vi "Normal to HEX string.vi"(1 "input normal string":string="0100") -> (0 "output HEX string":string)   [LabVIEW 2023]
panel:
  out "reversed":string
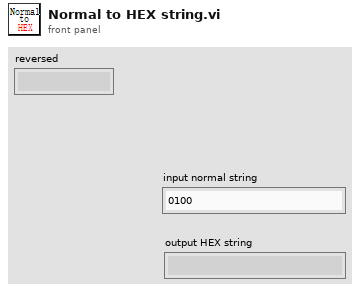
[diagram p1: front panel]
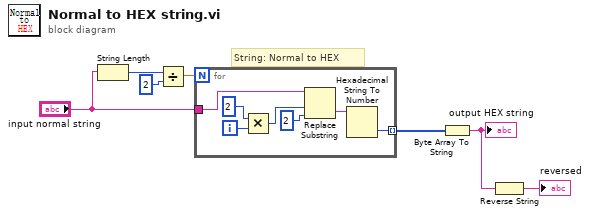
[diagram p0: block diagram]
diagram:
  # "String: Normal to HEX"
  n1 = String Length(string="input normal string") -> (length=w6:i32)
  n2 = Divide(x=w6, y=2) -> (x/y=w5:dbl)
  n3 = for {
    N: w5 -> [_]
    tunnel: "input normal string" -> [w14]
    tunnel: [w8] -> w7 mode=indexing
    i -> [w13]
    n4 = Multiply(x=2, y=w13) -> (x*y=w11:i32)
    n5 = Replace Substring(2:2 ("长度（子字符串长度）"), 3:w11, 5:w14) -> (0:w9:string)  [unwired: 1 in, 1 out]
    n6 = Hexadecimal String To Number(string=w9) -> (number=w8:u32)  [unwired: 2 in, 1 out]
  }
  n7 = Byte Array To String(unsigned byte array=w7) -> (string=w2:string)
  "output HEX string" <- w2
  n8 = Reverse String(1:w2) -> (0:→"reversed":string)
